vi "update offsets on disk.vi"(8 "error in (no error)":errorcluster, 10 "Offset IONames":string[](array[string]), 11 "Offset Values":dbl[](array[numeric])) -> (0 "error out":errorcluster)   [LabVIEW 2017, in "DAQ.lvclass"]
doc: "Developed by Kevin Thompson\nkevin@thompsonengineering.net\n\nCopyright 2018-2020\nThompson Engineering, LLC"
uses:
  DAQ.lvclass
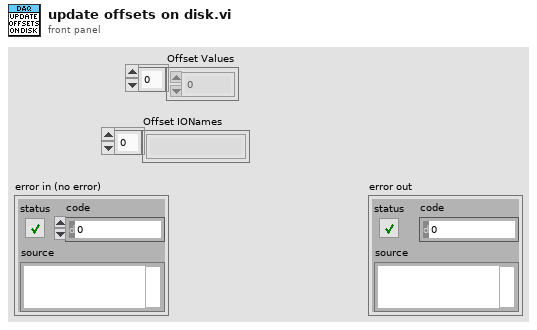
[diagram p1: front panel]
types:
  T1 = typedef "DAQ.lvclass/offsets cluster.ctl" = cluster{"Offset IONames":string[], "Offset Value":dbl[]}
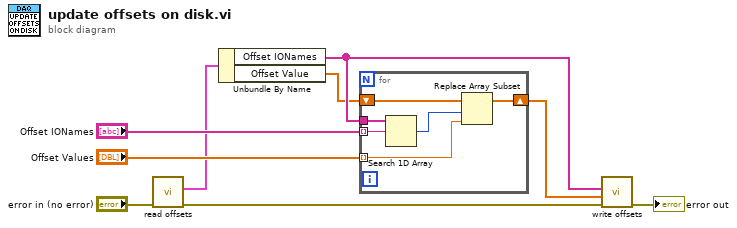
[diagram p0: block diagram]
diagram:
  n1 = call "read offsets.vi"("error in (no error)"="error in (no error)") -> ("error out"=w7:errorcluster, "offsets"=w1:T1)  [unwired: 9 in]
  n2 = Unbundle By Name(w1) -> ("Offset IONames"=w5:string[], "Offset Value"=w4:dbl[])
  n3 = for {
    tunnel: "Offset IONames" -> [w14] mode=indexing
    tunnel: "Offset Values" -> [w11] mode=indexing
    tunnel: w5 -> [w15]
    shift-right: [w10] -> w6
    shift-left: w4 -> [w13]
    n4 = Search 1D Array(1D array=w15, element=w14) -> (index of element=w12:i32)  [unwired: 1 in]
    n5 = Replace Array Subset(array=w13, new element=w11, index=w12) -> (w10:dbl[])
  }
  n6 = call "write offsets.vi"("error in (no error)"=w7, "Offset Value"=w6, "Offset IOName"=w5) -> ("error out"=→"error out":errorcluster)  [unwired: 7 in, 1 out]
